vi "Write Address.vi"(8 "error in (no error)":errorcluster, 10 "Address":refnum<visa-resource-name>="COM3", 11 "KH7008 in":refnum<class "Instrument.KH7008.lvclass">) -> (0 "error out":errorcluster, 3 "KH7008 out":refnum<class "Instrument.KH7008.lvclass">)   [LabVIEW 2016, in "Instrument.KH7008.lvclass"]
uses:
  Instrument.KH7008.lvclass
  Instrument.KH7008.lvclass/Instrument.KH7008.ctl
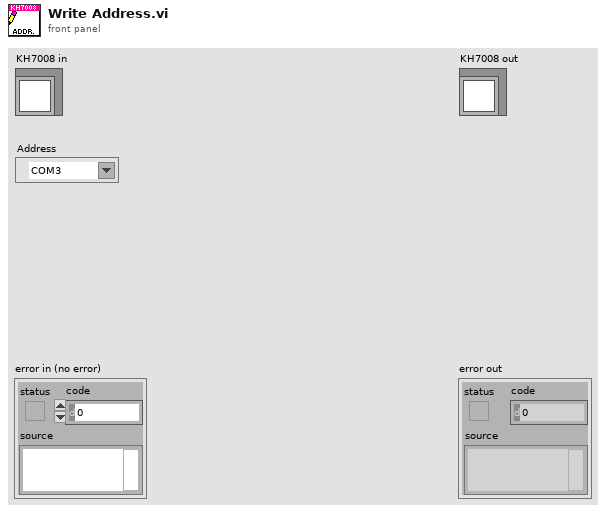
[diagram p1: front panel]
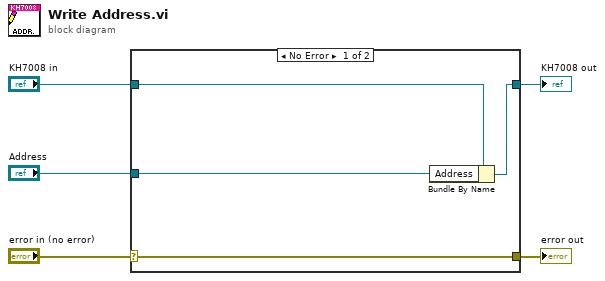
[diagram p0: block diagram]
diagram:
  n1 = case shown="No Error" "error in (no error)" {
    selector: "error in (no error)" -> [w9 w10]
    tunnel: [w9 w10] -> w4
    tunnel: [w7 w11] -> w2
    tunnel: "KH7008 in" -> [w8 w11]
    tunnel: "Address" -> [w6 _]
    frame No Error {
      n2 = Bundle By Name(cluster=w8, "Address"=w6) -> (w7:refnum<class "Instrument.KH7008.lvclass">)
    }
    frame Error {
    }
  }
  "error out" <- w4
  "KH7008 out" <- w2
